vi "Autonomous Independent.vi"() -> ()   [LabVIEW 2016]
doc: "This VI is called when autonomous begins, and will automatically be terminated when autonomous ends. You can carry out timed or sensor driven robot movement independently without needing to return to the caller."
uses:
  Auto/AutoModes.ctl
  Robot Global Data.vi
panel:
  out "error out":errorcluster
  in  "error in":errorcluster
  # "Be sure to right-click and choose Data Operations>>Make Current Value default if you want to save the array values with the VI"
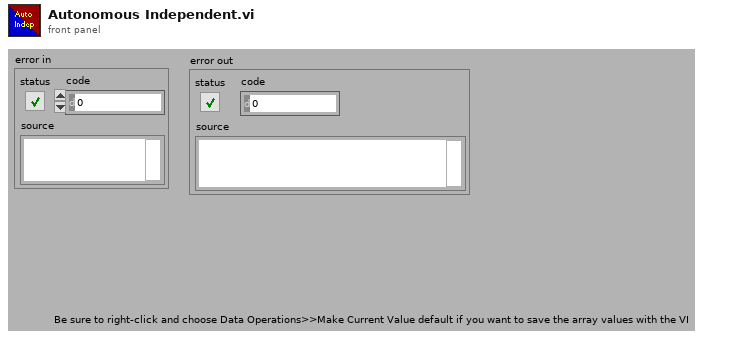
[diagram p1: front panel]
types:
  T1 = typedef "AutoModes.ctl" = enum16{"Do Nothing", "Cross Baseline", "Gear Front", "Gear Left", "Gear Right"}
  T2 = cluster{"X":dbl, "Y":dbl, "Z":dbl, "B (Straight Drive)":bool, "T1 (Climber Up)":bool, "T2 (Climber Down)":bool, "Pinky Trigger (Low Sensitivity Drive)":bool, "Trigger Full Press (Reverse Drive)":bool, "LED Green":bool}
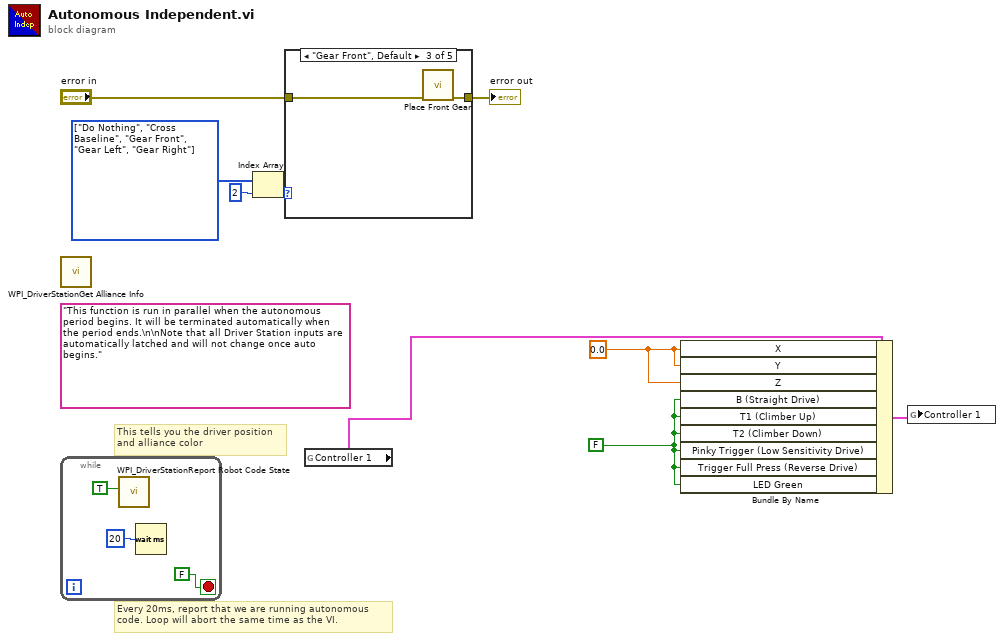
[diagram p0: block diagram]
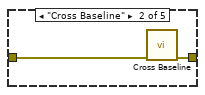
[diagram p3: hidden frame]
diagram:
  w1 = FALSE
  w2 = 0.0 ("X")
  (unwired) "This function is run in parallel when the autonomous period begins. It will be terminated automatically when the period ends.\n\nNote that all Driver Station inputs are automatically latched and will not change once auto begins."
  w7 = T1[] [enum."Do Nothing", enum."Cross Baseline", enum."Gear Front", enum."Gear Left", enum."Gear Right"] items=["Do Nothing", "Cross Baseline", "Gear Front", "Gear Left", "Gear Right"]
  # "Every 20ms, report that we are running autonomous\ncode. Loop will abort the same time as the VI."
  # "This tells you the driver position\nand alliance color"
  n1 = call <vilib>:"WPI_DriverStationGet Alliance Info.vi"() -> ()  [unwired: 12 out]
  n2 = while {
    stop <- FALSE stop-if-true
    n3 = call <vilib>:"WPI_DriverStationReport Robot Code State.vi"("Autonomous"=TRUE) -> ()  [unwired: 10 in, 1 out]
    n4 = Wait (ms)(milliseconds to wait=u32 20) -> ()  [unwired: 1 out]
  }
  n5 = Index Array(array=w7, index=2) -> (element=w6:T1)
  n6 = case shown="\"Gear Front\", Default" w6 {
    tunnel: "error in" -> [w13 w15 w17 w18 w19]
    tunnel: [w13 w14 w16 w18 w19] -> w8
    frame "Do Nothing" {
    }
    frame "Cross Baseline" {
      n7 = call "Cross Baseline.vi"("error in"=w15) -> ("error out"=w14:errorcluster)  [unwired: 9 in]
    }
    frame "Gear Front", Default {
      n8 = call "Place Front Gear.vi"("error in"=w17) -> ("error out"=w16:errorcluster)  [unwired: 10 in]
    }
    frame "Gear Left" {
    }
    frame "Gear Right" {
    }
  }
  "error out" <- w8
  n9 = global read "Robot Global Data.vi" "Controller 1"() -> (w4:T2)
  n10 = Bundle By Name(cluster=w4, "X"=w2, "Y"=w2, "Z"=w2, "B (Straight Drive)"=w1, "T1 (Climber Up)"=w1, "T2 (Climber Down)"=w1, "Pinky Trigger (Low Sensitivity Drive)"=w1, "Trigger Full Press (Reverse Drive)"=w1, "LED Green"=w1) -> (w3:T2)
  n11 = global write "Robot Global Data.vi" "Controller 1"(w3) -> ()
